vi "TCP-Grab String.vi"(0 "connection ID":refnum<k5>, 7 "No timeout?":bool, 11 "error in (no error)":errorcluster) -> (4 "connection ID out":refnum<k5>, 6 "data out":string, 15 "error out":errorcluster)   [LabVIEW 2020]
panel:
  out "Elapsed time (ms)":u32
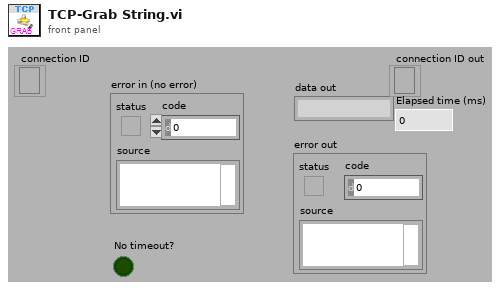
[diagram p1: front panel]
types:
  T1 = enum16{"Standard", "Buffered", "CRLF", "Immediate"}
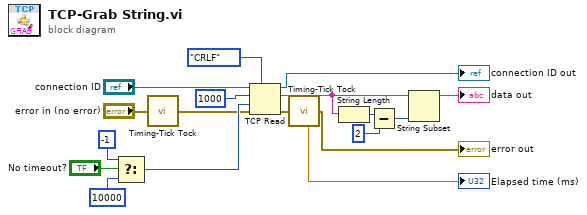
[diagram p0: block diagram]
diagram:
  n1 = Select(t=-1 ("timeout ms (25000)"), s="No timeout?", f=10000 ("timeout ms (25000)")) -> (s? t:f=w10:i32)
  n2 = call "Timing-Tick Tock.vi"("error in (no error)"="error in (no error)") -> ("error out"=w8:errorcluster)  [unwired: 5 in, 1 out]
  n3 = TCP Read(connection ID="connection ID", bytes to read=1000, error in (no error)=w8, 7:T1."CRLF" ("mode (standard)"), 9:w10) -> (connection ID out=→"connection ID out":refnum<k5>, data out=w3:string, error out=w18:errorcluster)
  n4 = call "Timing-Tick Tock.vi"("error in (no error)"=w18) -> ("Elapsed time (ms)"=→"Elapsed time (ms)":dbl, "error out"=→"error out":errorcluster)  [unwired: 5 in]
  n5 = String Length(string=w3) -> (length=w4:i32)
  n6 = Subtract(x=w4, y=2) -> (x-y=w2:i32)
  n7 = String Subset(string=w3, length (rest)=w2) -> (substring=→"data out":string)  [unwired: 1 in]
